vi "Switch Obs Lat and Long.vi"(11 "Obstacle Lats and Longs for GIC":T2) -> (3 "Obstacle Lats and Longs switched":T1)   [LabVIEW 2014]
panel:
  # "Switch Lat and Long arrays in Obstacle cluster for graph"
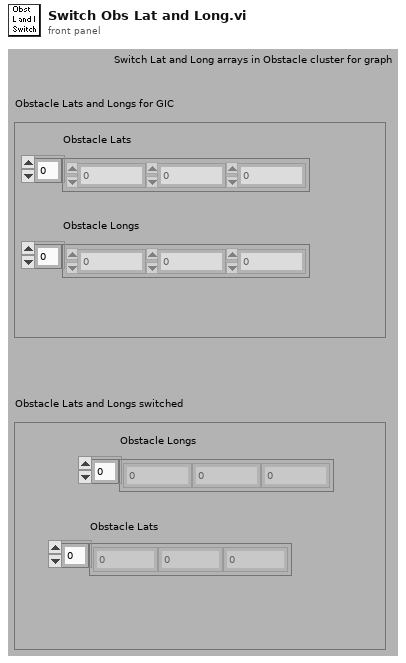
[diagram p1: front panel]
types:
  T1 = cluster{"Obstacle Longs":dbl[], "Obstacle Lats":dbl[]}
  T2 = cluster{"Obstacle Lats":dbl[], "Obstacle Longs":dbl[]}
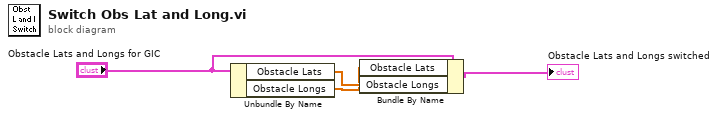
[diagram p0: block diagram]
diagram:
  n1 = Unbundle By Name("Obstacle Lats and Longs for GIC") -> ("Obstacle Lats"=w3:dbl[], "Obstacle Longs"=w2:dbl[])
  n2 = Bundle By Name(cluster="Obstacle Lats and Longs for GIC", "Obstacle Lats"=w2, "Obstacle Longs"=w3) -> (→"Obstacle Lats and Longs switched":T2)
